vi "global 4.vi"() -> ()   [LabVIEW 2015]
panel:
  out "global set packet data out":u8[](array[numeric])
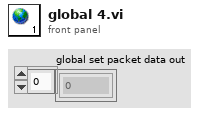
[diagram p1: front panel]
diagram:
